vi "Pcre2CompileError.vi"(8 "error in":errorcluster, 9 "ErrorOffset":u64, 10 "ErrorCode":i32, 11 "pCode":u64 format="%.0x") -> (0 "error out":errorcluster, 3 "pCode":u64 format="%.0x")   [LabVIEW 2021, in "libpcre2-8.lvlib"]
uses:
  libpcre2-8.lvlib
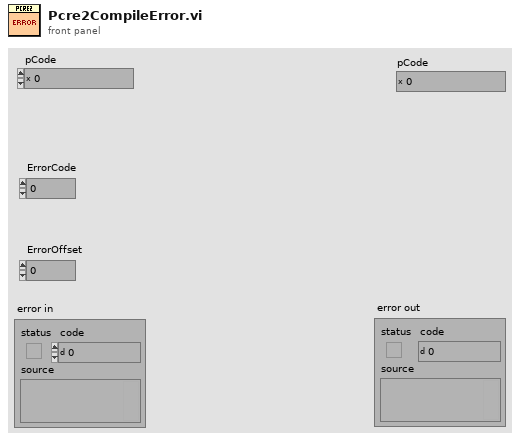
[diagram p1: front panel]
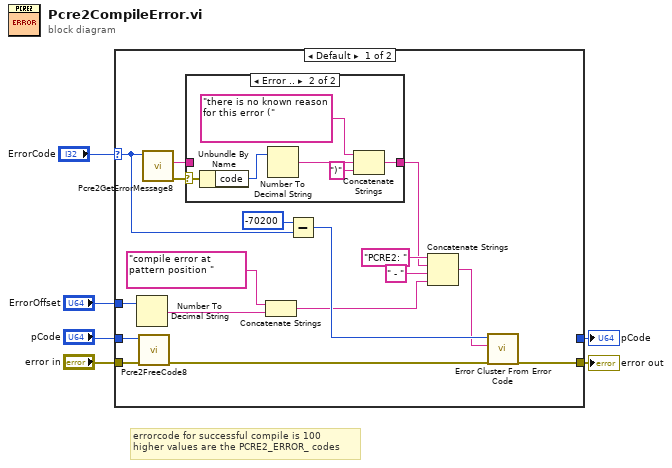
[diagram p0: block diagram]
diagram:
  # "errorcode for successful compile is 100\nhigher values are the PCRE2_ERROR_ codes"
  n1 = case shown="Default" "ErrorCode" {
    selector: "ErrorCode" -> [w15 _]
    tunnel: "error in" -> [w20 w32]
    tunnel: [w14 w32] -> w3
    tunnel: [_ w31] -> w4
    tunnel: "pCode" -> [w19 w31]
    tunnel: "ErrorOffset" -> [w21 _]
    frame Default {
      n2 = Number To Decimal String(number=w21) -> (decimal integer string=w23:string)  [unwired: 1 in]
      n3 = call "Pcre2FreeCode8.vi"("error in"=w20, "pCode"=w19) -> ("error out"=w13:errorcluster)  [unwired: 9 in]
      n4 = call "Pcre2GetErrorMessage8.vi"("ErrorCode"=w15) -> ("error out"=w17:errorcluster, "ErrorMessage"=w18:string)  [unwired: 8 in, 1 out]
      n5 = case shown="Error .." w17 {
        selector: w17 -> [_ w26]
        tunnel: w18 -> [w24 _]
        tunnel: [w24 w30] -> w9
        frame No Error {
        }
        frame Error {
          n6 = Unbundle By Name(w26) -> ("code"=w25:i32)
          n7 = Number To Decimal String(number=w25) -> (decimal integer string=w28:string)  [unwired: 1 in]
          n8 = Concatenate Strings("there is no known reason for this error (" ("ErrorMessage"), w28, ")" ("string")) -> (w30:string)
        }
      }
      n9 = Concatenate Strings("compile error at pattern position " ("string"), w23) -> (w7:string)
      n10 = Subtract(x=-70200 ("errorcode"), y=w15) -> (x-y=w12:i32)
      n11 = Concatenate Strings("PCRE2: " ("string"), w9, " - " ("string"), w7) -> (w8:string)
      n12 = call <vilib>:"Error Cluster From Error Code.vi"("error in (no error)"=w13, "error message (\"\")"=w8, "error code (0)"=w12) -> ("error out"=w14:errorcluster)  [unwired: 6 in]
    }
    frame 100 {
    }
  }
  "error out" <- w3
  "pCode" <- w4
